vi "Test - 2's Complement.vi"() -> ()   [LabVIEW 2021]
panel:
  in  "stop":bool
  in  "High":bool[](array[boolean])
  in  "Low":bool[](array[boolean])
  out "Output I16":i16
  out "Reversed Bool":bool[](array[boolean])
  out "L Bool":bool[](array[boolean])
  out "H Bool":bool[](array[boolean])
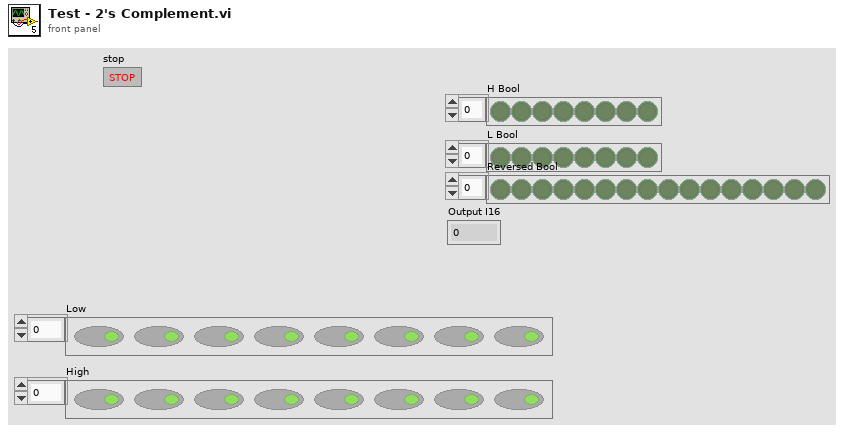
[diagram p1: front panel]
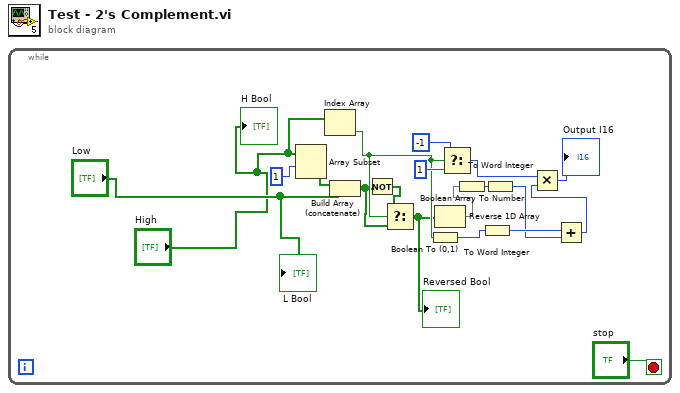
[diagram p0: block diagram]
diagram:
  n1 = while {
    stop <- "stop" stop-if-true
    n2 = Array Subset(array="High", index=1) -> (w19:bool[])  [unwired: 1 in]
    n3 = Index Array(array="High") -> (element=w10:bool)  [unwired: 1 in]
    n4 = Build Array (concatenate)(w19, "Low") -> (w8:bool[])
    n5 = Not(x=w8) -> (.not. x?=w9:bool[])
    n6 = Select(t=w9, s=w10, f=w8) -> (s? t:f=w5:bool[])
    "Reversed Bool" <- w5
    n7 = Boolean To (0,1)(Boolean=w10) -> (0, 1=w12:i16)
    n8 = Reverse 1D Array(array=w5) -> (reversed array=w4:bool[])
    n9 = Select(t=i16 -1, s=w10, f=i16 1) -> (s? t:f=w16:i16)
    n10 = Boolean Array To Number(Boolean array=w4) -> (number=w17:u32)
    n11 = To Word Integer(number=w12) -> (16bit integer=w11:i16)
    n12 = To Word Integer(number=w17) -> (16bit integer=w7:i16)
    n13 = Add(x=w11, y=w7) -> (x+y=w6:i16)
    n14 = Multiply(x=w16, y=w6) -> (x*y=→"Output I16":i16)
    "H Bool" <- "High"
    "L Bool" <- "Low"
  }
